vi "Make_Origin_Zero-1.vi"(4 "[IN] # Track":i32, 5 "[IN] Dot Statuses":i16[][](array[numeric]), 6 "[IN] Start Pos":i32[](array[numeric]), 7 "[IN] Tracks":dbl[][](array[numeric])) -> (1 "[OUT] Statuses":i16[][](array[numeric]), 2 "[OUT] Start Pos":i32[](array[numeric]), 3 "[OUT] Tracks":dbl[][](array[numeric]))   [LabVIEW 2013]
doc: "This subVI deletes the initial point as the fake origin"
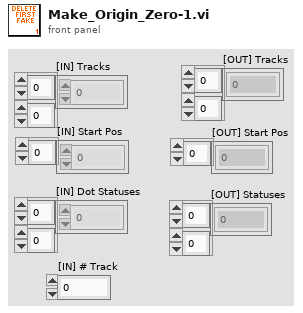
[diagram p1: front panel]
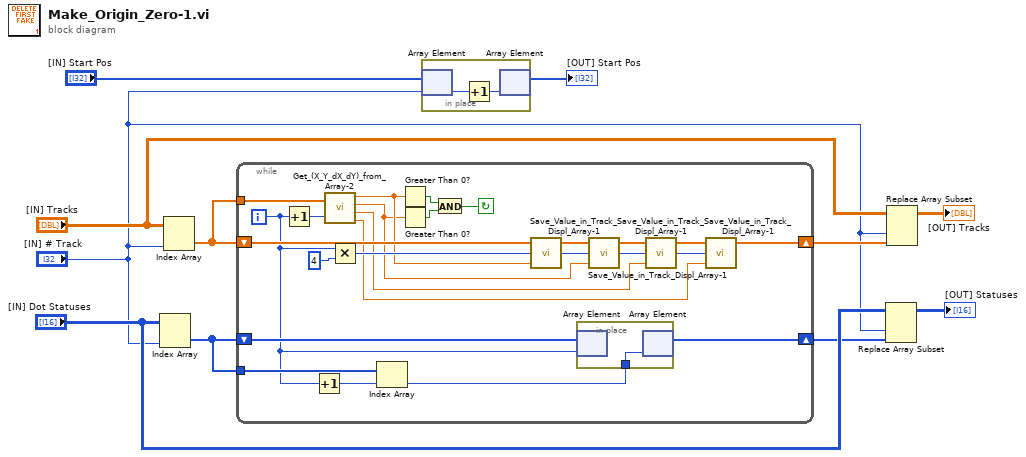
[diagram p0: block diagram]
diagram:
  n1 = Index Array(array="[IN] Dot Statuses", index (col)="[IN] # Track") -> (element=w6:i16[])  [unwired: 1 in]
  n2 = Index Array(array="[IN] Tracks", index (col)="[IN] # Track") -> (element=w11:dbl[])  [unwired: 1 in]
  n3 = while {
    shift-right: [w25] -> w7
    shift-left: w11 -> [w34]
    tunnel: w11 -> [w36]
    shift-right: [w21] -> w4
    shift-left: w6 -> [w24]
    tunnel: w6 -> [w23]
    i -> [w20]
    stop <- w18 continue-if-true
    n4 = Increment(x=w20) -> (x+1=w35:i32)
    n5 = Increment(x=w20) -> (x+1=w19:i32)
    n6 = call "Get_(X_Y_dX_dY)_from_Array-2.vi"("(X,Y,dX,dY)"=w36, "Index of Displacement"=w35) -> ("X"=w29:dbl, "Y"=w28:dbl, "dX"=w27:dbl, "dY"=w26:dbl)
    n7 = Multiply(x=w20, y=4) -> (x*y=w32:i32)
    n8 = Index Array(array=w23, index=w19) -> (element=w22:i16)
    n9 = Greater Than 0?(x=w29) -> (x > 0?=w31:bool)
    n10 = Greater Than 0?(x=w28) -> (x > 0?=w30:bool)
    n11 = And(x=w31, y=w30) -> (x .and. y?=w18:bool)
    n12 = call "Save_Value_in_Track_Displ_Array-1.vi"("[IN] Value"=w29, "[IN] Index"=w32, "[IN] Empty tracks\nfor points saving"=w34) -> ("[OUT] Index ++"=w16:i32, "[OUT Track with saved value"=w17:dbl[])  [unwired: 1 in]
    n13 = in-place {
      in-place-border: w22 -> [w37]
      n14 = in-place-array #1(w24, w20) -> ()  [unwired: 1 out]
      n15 = in-place-array #1(w37) -> (w21:i16[])  [unwired: 1 out]
    }
    n16 = call "Save_Value_in_Track_Displ_Array-1.vi"("[IN] Value"=w28, "[IN] Index"=w16, "[IN] Empty tracks\nfor points saving"=w17) -> ("[OUT] Index ++"=w14:i32, "[OUT Track with saved value"=w15:dbl[])  [unwired: 1 in]
    n17 = call "Save_Value_in_Track_Displ_Array-1.vi"("[IN] Value"=w27, "[IN] Index"=w14, "[IN] Empty tracks\nfor points saving"=w15) -> ("[OUT] Index ++"=w12:i32, "[OUT Track with saved value"=w13:dbl[])  [unwired: 1 in]
    n18 = call "Save_Value_in_Track_Displ_Array-1.vi"("[IN] Value"=w26, "[IN] Index"=w12, "[IN] Empty tracks\nfor points saving"=w13) -> ("[OUT Track with saved value"=w25:dbl[])  [unwired: 1 in, 1 out]
  }
  n19 = in-place {
    n20 = in-place-array #2("[IN] Start Pos", "[IN] # Track") -> (w39:i32)
    n21 = Increment(x=w39) -> (x+1=w38:i32)
    n22 = in-place-array #2(w38) -> (→"[OUT] Start Pos":i32[])  [unwired: 1 out]
  }
  n23 = Replace Array Subset(array="[IN] Dot Statuses", new element=w4, index (col)="[IN] # Track") -> (→"[OUT] Statuses":i16[][])  [unwired: 1 in]
  n24 = Replace Array Subset(array="[IN] Tracks", new element=w7, index (col)="[IN] # Track") -> (→"[OUT] Tracks":dbl[][])  [unwired: 1 in]
